vi "Get Keys Mapping.vi"() -> (0 "Keys Mapping":map{string, string}(c390))   [LabVIEW 2021, in "Seq Edit Quick Drop.lvlib"]
uses:
  Seq Edit Quick Drop.lvlib
  Scan Codes Mapping.vi
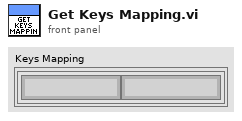
[diagram p1: front panel]
types:
  T1 = typedef "Seq Edit Quick Drop.lvlib/Key Code.ctl" = cluster{"Key":string, "Scan Code":i16}
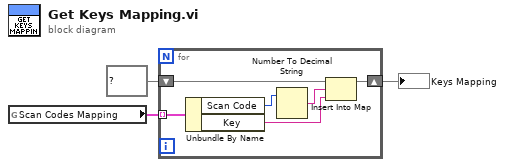
[diagram p0: block diagram]
diagram:
  n1 = global read "Scan Codes Mapping.vi" "Scan Codes Mapping"() -> (w3:T1[])
  n2 = for {
    tunnel: w3 -> [w9] mode=indexing
    shift-right: [w6] -> w1
    shift-left: map{string, string} {} ("Size: 0") -> [w5]
    n3 = Unbundle By Name(w9) -> ("Scan Code"=w7:i16, "Key"=w8:string)
    n4 = Number To Decimal String(number=w7) -> (decimal integer string=w4:string)  [unwired: 1 in]
    n5 = Insert Into Map(map in=w5, key=w4, value=w8) -> (map out=w6:map{string, string})  [unwired: 2 out]
  }
  "Keys Mapping" <- w1
